vi "Fetch Multiple Record Single Channel (DBL).vi"(5 "FIFO Type":enum16{"FPGA to Host FIFO (U64)", "Generic"}(ring), 7 "Timeout (s)":i32=5, 8 "error in":errorcluster, 10 "Records to Fetch":i32, 11 "FPGA VI Reference In":refnum<k20>) -> (0 "error out":errorcluster, 2 "Acquired Data":dbl[][](array[numeric]) format="%.2f", 3 "FPGA VI Reference Out":refnum<k20>, 4 "Elements Remaining":u32)   [LabVIEW 2011]
uses:
  <userlib>/FlexRIO Host Library/FlexRIO Host API/Acquire/Fetch/Fetch Acquired Data (U64).vi
  <vilib>/Utility/error.llb/Error Cluster From Error Code.vi
  <vilib>/rvi/errors/niLvFpgaAdjustHostInterfaceError.vi
  <vilib>/rvi/interface/nirviReadWriteControl/nirviReadWriteControl.xnode
  NiFpgaLv.dll
  <vilib>/rvi/interface/Simulation/niFpgaSimulationCallBeginRW.vi
  <userlib>/FlexRIO Host Library/FlexRIO Host Library (User).lvlib
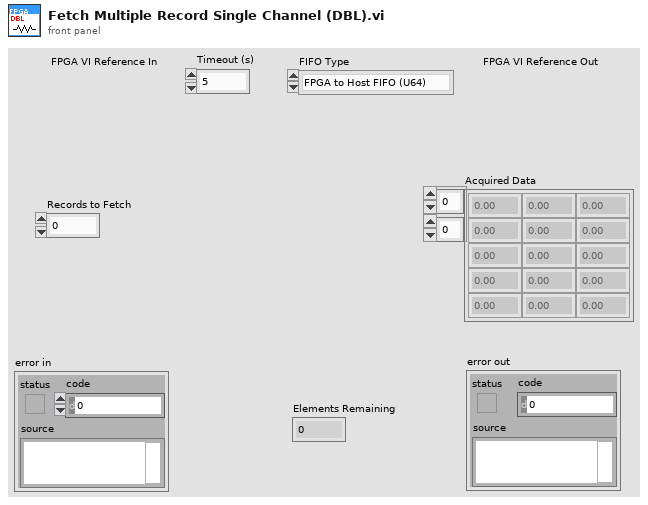
[diagram p1: front panel]
types:
  T1 = cluster{"Load Record Parameters?":bool, "Pre Trigger Samples":u16, "Samples per Record":u16, "Trigger Hold Off":u16, "Record Count":u16}
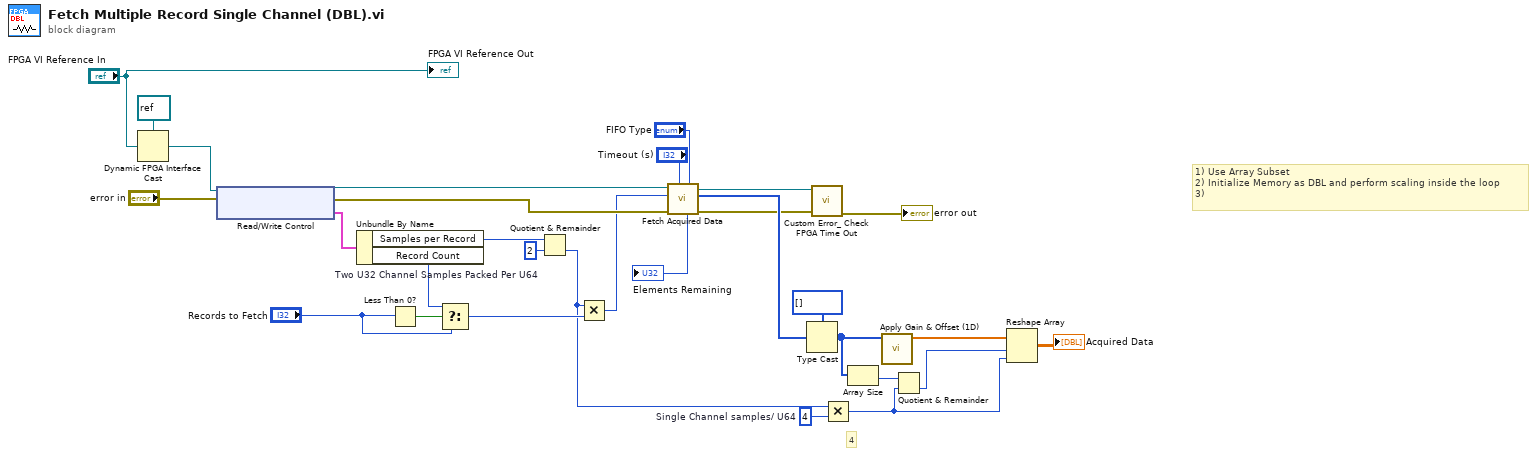
[diagram p0: block diagram]
diagram:
  w3 = u16 2  # Two U32 Channel Samples Packed Per U64
  w14 = u16 4  # Single Channel samples/ U64
  # "4"
  # "1) Use Array Subset\n2) Initialize Memory as DBL and perform scaling inside the loop\n3)"
  n1 = Dynamic FPGA Interface Cast(Session In=refnum<k20> refnum ("Type"), Type="FPGA VI Reference In") -> (Session Out=w27:refnum<k20>)
  n2 = xnode "Read/Write Control"("FPGA VI Reference In"=w27, "error in"="error in") -> ("FPGA VI Reference Out"=w22:refnum<k20>, "error out"=w21:errorcluster, "Record Parameters"=w26:T1)
  n3 = Unbundle By Name(w26) -> ("Samples per Record"=w4:u16, "Record Count"=w24:u16)
  n4 = Less Than 0?(x="Records to Fetch") -> (x < 0?=w25:bool)
  n5 = Select(t=w24, s=w25, f="Records to Fetch") -> (s? t:f=w15:i32)
  n6 = Quotient & Remainder(x=w4, y=w3) -> (floor(x/y)=w5:u16)  [unwired: 1 out]
  n7 = Multiply(x=w5, y=w15) -> (x*y=w10:i32)
  n8 = call-poly <userlib>:"Fetch Acquired Data.vi"("FIFO Type"="FIFO Type", "Timeout (s)"="Timeout (s)", "error out"=w21, "Samples"=w10, "FPGA VI Reference In"=w22) -> ("error out"=w12:errorcluster, "Data"=w18:u64[], "FPGA VI Reference Out"=w13:refnum<k20>, "Elements Remaining"=→"Elements Remaining":u32)  [unwired: 3 in]
  n9 = Type Cast(type=i16[] [], x=w18) -> (*(type *) &x=w2:i16[])
  n10 = call <userlib>:"Custom Error_ Check FPGA Time Out.vi"("error in"=w12, "FPGA VI Reference In"=w13) -> ("error out"=→"error out":errorcluster)  [unwired: 8 in, 1 out]
  n11 = Multiply(x=w5, y=w14) -> (x*y=w8:u16)
  n12 = Array Size(array=w2) -> (size(s)=w9:i32)
  n13 = call <userlib>:"Apply Gain & Offset (1D).vi"("Raw Data"=w2) -> ("Scaled Data"=w1:dbl[])  [unwired: 10 in]
  n14 = Quotient & Remainder(x=w9, y=w8) -> (floor(x/y)=w7:i32)  [unwired: 1 out]
  n15 = Reshape Array(w1, w7, w8) -> (→"Acquired Data":dbl[][])
  "FPGA VI Reference Out" <- "FPGA VI Reference In"
